vi "Focus Close.vi"(8 "error in (no error)":errorcluster, 11 "NewFocus in":refnum<class "NewFocus.lvclass">) -> (0 "error out":errorcluster, 3 "NewFocus out":refnum<class "NewFocus.lvclass">)   [LabVIEW 2024, in "NewFocus.lvclass"]
uses:
  NewFocus.lvclass
  NewFocus.lvclass/NewFocus.ctl
  Focus Class/Focus Class.lvclass
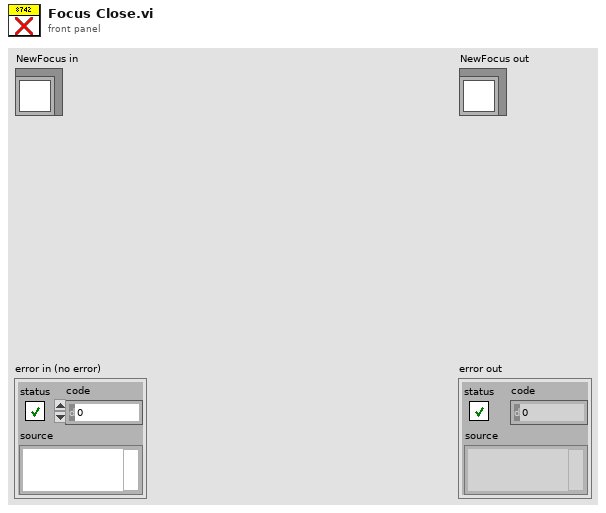
[diagram p1: front panel]
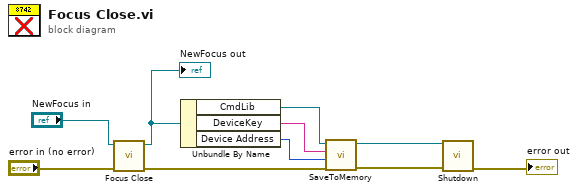
[diagram p0: block diagram]
diagram:
  n1 = call-parent "Focus Close.vi"("error in (no error)"="error in (no error)", "Focus Class in"="NewFocus in") -> ("error out"=w6:errorcluster, "Focus Class out"=w8:refnum<class "NewFocus.lvclass">)  [unwired: 8 in]
  "NewFocus out" <- w8
  n2 = Unbundle By Name(w8) -> ("CmdLib"=w4:refnum<k24>, "DeviceKey"=w2:string, "Device Address"=w1:i32)
  n3 = call "SaveToMemory.vi"("error in (no error)"=w6, "Device Address In"=w1, "DeviceKey In"=w2, "CmdLib In"=w4) -> ("error out"=w5:errorcluster, "CmdLib Out"=w3:refnum<k24>)  [unwired: 2 out]
  n4 = call "Shutdown.vi"("error in (no error)"=w5, "CmdLib In"=w3) -> ("error out"=→"error out":errorcluster)  [unwired: 4 in, 1 out]
